vi "NewSeccion.vi"(10 "Rectangle":T1 {"Rotation" format="%.2f"; "Left" scale=0.0..1024.0; "Right" scale=0.0..1024.0}, 11 "Refnum in":T2) -> (1 "Rojo":bool, 2 "Azul":bool, 3 "Verde":bool, 4 "Amarillo":bool, 5 "Color Spectrum":dbl[](array[numeric]), 6 "Negro":bool)   [LabVIEW 2018]
uses:
  <vilib>/vision/Image Controls.llb/IMAQ Image.ctl
  <vilib>/vision/NI_Vision_Development_Module.lvlib
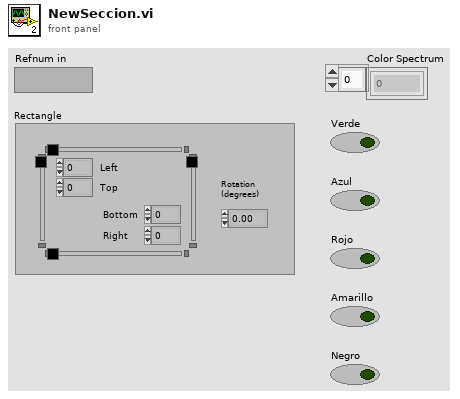
[diagram p1: front panel]
types:
  T1 = typedef "IMAQ Rectangle" = cluster{"Left":i32, "Top":i32, "Right":i32, "Bottom":i32, "Rotation":dbl}
  T2 = typedef "IMAQ Image.ctl" = refnum<image>
  T3 = typedef "ROI Descriptor" = cluster{"Global Rectangle":i32[], "Contours":cluster{"ID":enum32{"External", "Internal"}, "Type":u32, "Coordinates":i32[]}[]}
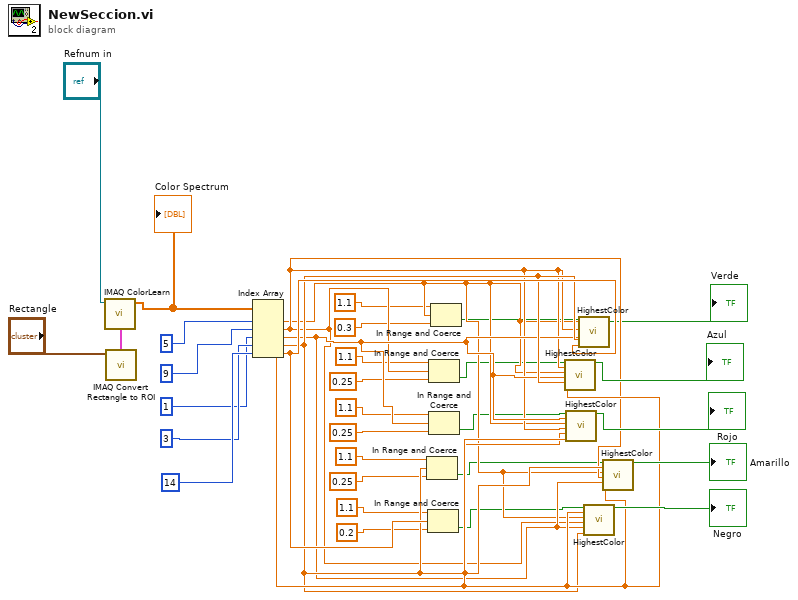
[diagram p0: block diagram]
diagram:
  n1 = call "IMAQ Convert Rectangle to ROI"("Rectangle"="Rectangle") -> ("ROI Descriptor"=w2:T3)  [unwired: 8 in, 1 out]
  n2 = call "IMAQ ColorLearn"("ROI Descriptor"=w2, "Image"="Refnum in") -> ("Color Spectrum"=w9:dbl[])  [unwired: 6 in, 1 out]
  "Color Spectrum" <- w9
  n3 = Index Array(array=w9, index #1=5 ("index"), index #2=9 ("index"), index #3=1 ("index"), index #4=3 ("index"), index #5=14 ("index")) -> (element #1=w26:dbl, element #2=w27:dbl, element #3=w28:dbl, element #4=w29:dbl, element #5=w30:dbl)
  n4 = In Range and Coerce(upper limit=1.1, x=w29, lower limit=0.25) -> (In Range?=w24:bool)  [unwired: 1 out]
  n5 = In Range and Coerce(upper limit=1.1, x=w30, lower limit=0.2) -> (In Range?=w25:bool)  [unwired: 1 out]
  n6 = In Range and Coerce(upper limit=1.1, x=w27, lower limit=0.25) -> (In Range?=w22:bool)  [unwired: 1 out]
  n7 = In Range and Coerce(upper limit=1.1, x=w28, lower limit=0.25) -> (In Range?=w23:bool)  [unwired: 1 out]
  n8 = In Range and Coerce(upper limit=1.1, x=w26, lower limit=0.3) -> (In Range?=w21:bool)  [unwired: 1 out]
  n9 = call "HighestColor.vi"("Rango"=w22, "ColorPrincipal"=w27, "Color 1"=w26, "Color 2"=w28, "Color 3"=w29, "Color 4"=w30) -> ("Resultado"=→"Azul":bool)  [unwired: 13 in]
  n10 = call "HighestColor.vi"("Rango"=w23, "ColorPrincipal"=w28, "Color 1"=w26, "Color 2"=w27, "Color 3"=w29, "Color 4"=w30) -> ("Resultado"=→"Rojo":bool)  [unwired: 13 in]
  n11 = call "HighestColor.vi"("Rango"=w21, "ColorPrincipal"=w26, "Color 1"=w27, "Color 2"=w28, "Color 3"=w29, "Color 4"=w30) -> ("Resultado"=→"Verde":bool)  [unwired: 13 in]
  n12 = call "HighestColor.vi"("Rango"=w25, "ColorPrincipal"=w30, "Color 1"=w26, "Color 2"=w27, "Color 3"=w28, "Color 4"=w29) -> ("Resultado"=→"Negro":bool)  [unwired: 13 in]
  n13 = call "HighestColor.vi"("Rango"=w24, "ColorPrincipal"=w29, "Color 1"=w26, "Color 2"=w27, "Color 3"=w28, "Color 4"=w30) -> ("Resultado"=→"Amarillo":bool)  [unwired: 13 in]
